vi "about.vi"() -> ()   [LabVIEW 2011]
uses:
  <vilib>/Platform/browser.llb/Open URL in Default Browser (string).vi
panel:
  in  "Cancel Button":bool
  in  "issue 2":bool
  in  "issue":bool
  # "Software created by Johannes Rebling, summer 2012"
  # "Please report bugs and suggestions to:\njohannesrebling@gmail.com \nor report and issue on github!"
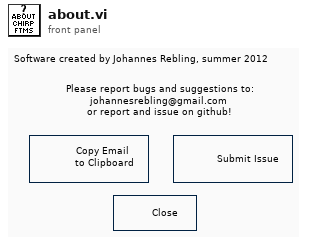
[diagram p1: front panel]
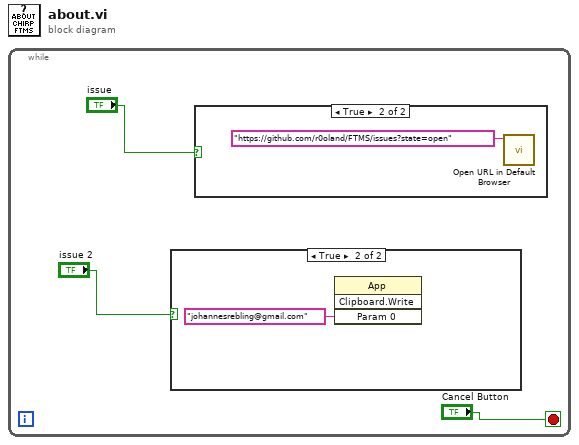
[diagram p0: block diagram]
diagram:
  n1 = while {
    stop <- "Cancel Button" stop-if-true
    n2 = case shown="True" "issue 2" {
      frame False {
      }
      frame True {
        n3 = invoke class="App" method="Clipboard.Write"("Param 0"="johannesrebling@gmail.com" ("Text")) -> ()  [unwired: 3 in, 4 out]
      }
    }
    n4 = case shown="True" "issue" {
      frame False {
      }
      frame True {
        n5 = call-poly <vilib>:"Open URL in Default Browser.vi"("URL"="https://github.com/r0oland/FTMS/issues?state=open") -> ()  [unwired: 5 in, 2 out]
      }
    }
  }
